vi "calcDistance.vi"(0 "currentPos x":dbl, 1 "currentPos y":dbl, 2 "currentPos z":dbl, 3 "savedPos x":dbl, 4 "savedPos y":dbl, 5 "savedPos z":dbl) -> (17 "Numeric":dbl)   [LabVIEW 2017]
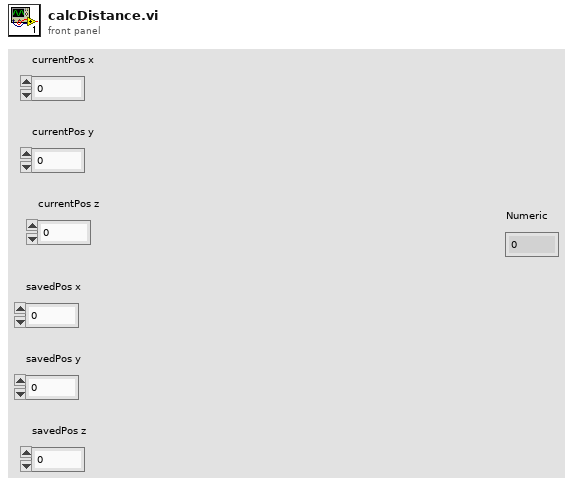
[diagram p1: front panel]
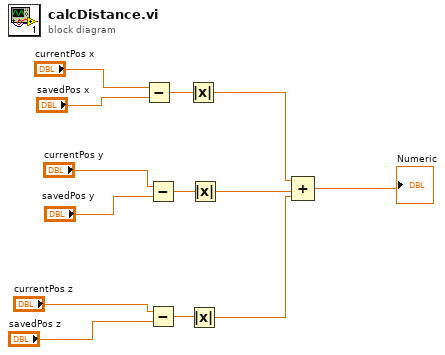
[diagram p0: block diagram]
diagram:
  n1 = Subtract(x="currentPos x", y="savedPos x") -> (x-y=w7:dbl)
  n2 = Subtract(x="currentPos y", y="savedPos y") -> (x-y=w5:dbl)
  n3 = Subtract(x="currentPos z", y="savedPos z") -> (x-y=w6:dbl)
  n4 = Absolute Value(x=w7) -> (abs(x)=w4:dbl)
  n5 = Absolute Value(x=w6) -> (abs(x)=w2:dbl)
  n6 = Absolute Value(x=w5) -> (abs(x)=w3:dbl)
  n7 = Compound Arithmetic op=ADD(w4, w3, w2) -> (→"Numeric":dbl)
